vi "Get Device Waveforms.vi"(8 "error in (no error)":errorcluster, 10 "AOwfm":waveform(dbl)[](array[waveform]), 11 "Channel Map":T2[](array[typedef])) -> (0 "error out":errorcluster, 2 "Device Waveforms":T1(array[cluster]))   [LabVIEW 2019, in "DAQmx.lvclass"]
uses:
  DAQmx.lvclass
  typedefs/DAQmx.Channel Map--Cluster.ctl
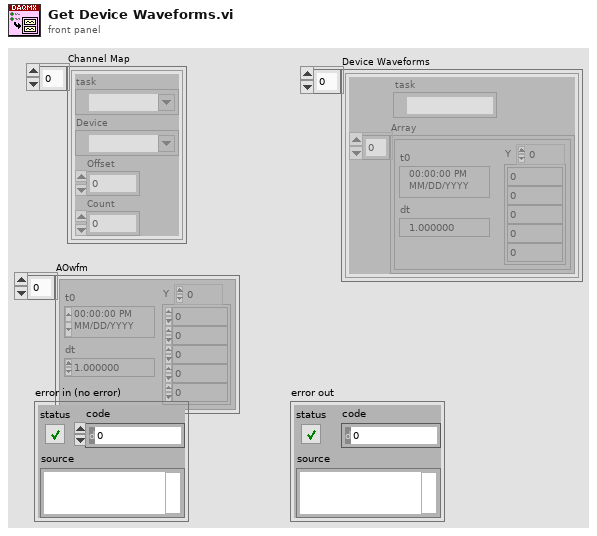
[diagram p1: front panel]
types:
  T1 = cluster{"task":refnum<k21>, "Array":waveform(dbl)[]}[]
  T2 = typedef "DAQmx.lvclass/DAQmx.Channel Map--Cluster.ctl" = cluster{"task":refnum<k21>, "Device":tag, "Offset":u32, "Count":u32}
  T3 = cluster{"task":refnum<k21>, "Array":waveform(dbl)[]}
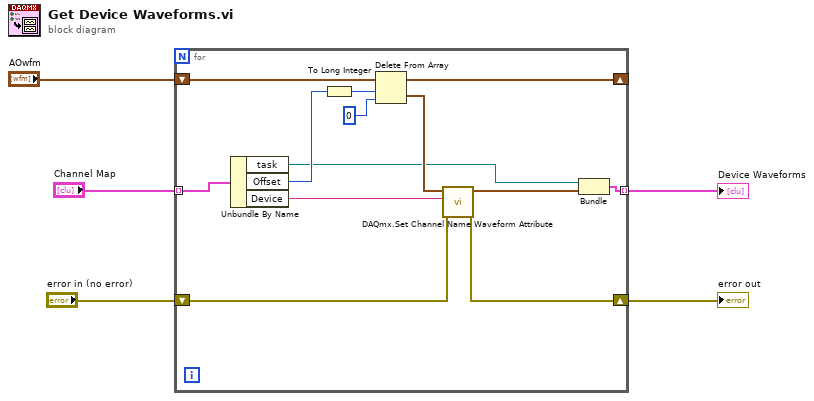
[diagram p0: block diagram]
diagram:
  n1 = for {
    shift-right: [w9] -> _
    shift-left: "AOwfm" -> [w14]
    tunnel: "Channel Map" -> [w13] mode=indexing
    tunnel: [w12] -> w1 mode=indexing
    shift-right: [w10] -> w5
    shift-left: "error in (no error)" -> [w11]
    n2 = Unbundle By Name(w13) -> ("task"=w6:refnum<k21>, "Offset"=w8:u32, "Device"=w7:tag)
    n3 = To Long Integer(number=w8) -> (32bit integer=w15:i32)
    n4 = Delete From Array(array=w14, length=w15, index=0) -> (deleted portion=w17:waveform(dbl)[], array with subset deleted=w9:waveform(dbl)[])
    n5 = call "DAQmx.Set Channel Name Waveform Attribute.vi"("error in (no error)"=w11, "DAQmx Device Name"=w7, "AOwfm"=w17) -> ("error out"=w10:errorcluster, "Array"=w16:waveform(dbl)[])  [unwired: 7 in]
    n6 = Bundle("task"=w6, "Array"=w16) -> (w12:T3)  [unwired: 1 in]
  }
  "error out" <- w5
  "Device Waveforms" <- w1
